vi "Start Logger.vi"(8 "error in (no error)":errorcluster, 11 "Worker in":refnum<class "Worker Actor.lvclass">) -> (0 "error out":errorcluster, 1 "tdms stream out":refnum<k34>, 2 "File Path":path, 3 "Worker out":refnum<class "Worker Actor.lvclass">)   [LabVIEW 2021, in "Worker Actor.lvclass"]
uses:
  Worker Actor.lvclass
  C:/GitHub/LabActor/Template Module/Template Module.lvclass
  Template Module/Template Module.lvclass/Template Module.ctl
  Worker Actor.lvclass/Worker Actor.ctl
  Loggers/Logger/Logger.lvclass/Logger.ctl
  NHMFL_Core/Libraries/File/File Class/File.lvclass/File.ctl
  Template Module/Read Logger.vi
  Read File prefix.vi
  Read Index digits.vi
  Loggers/Logger/Read File.lvclass.vi
  NHMFL_Core/Libraries/File/File Class/Write File Prefix.vi
  NHMFL_Core/Libraries/File/File Class/Write Index digits.vi
  NHMFL_Core/Libraries/File/File Class/Write Root Data Folder.vi
  Loggers/Logger/Write File.lvclass.vi
  Write File Path.vi
  Template Module/Write Logger.vi
  Read Use buffered logger.vi
  Loggers/Logger/Logger.lvclass
  NHMFL_Core/Libraries/File/Metadata/Metadata.lvclass
  NHMFL_Core/Libraries/File/File Class/File.lvclass
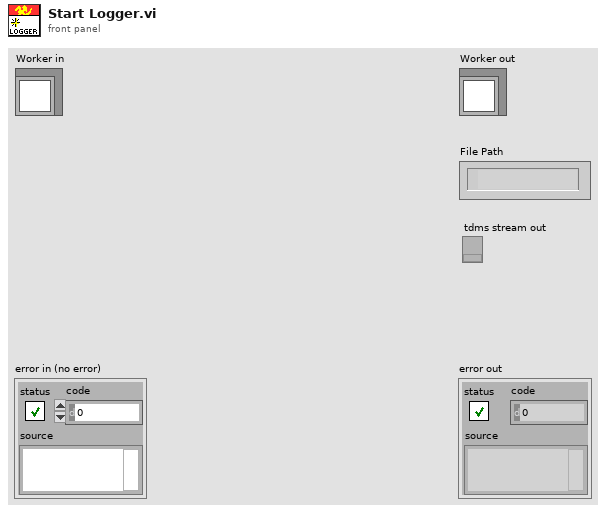
[diagram p1: front panel]
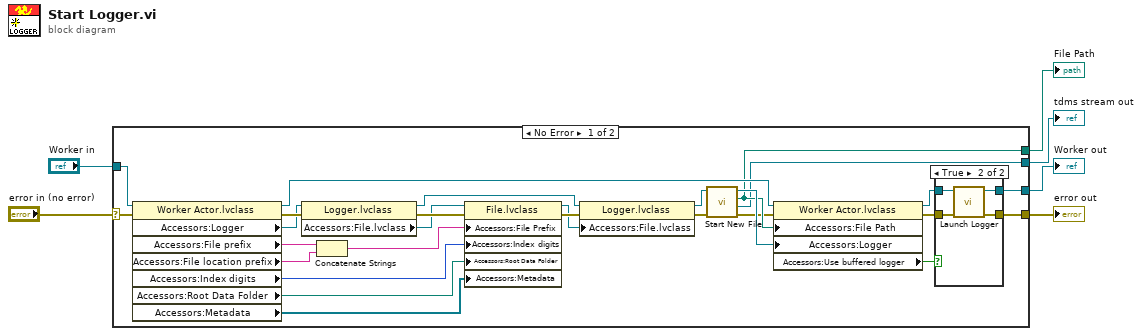
[diagram p0: block diagram]
diagram:
  n1 = case shown="No Error" "error in (no error)" {
    selector: "error in (no error)" -> [w31 w41]
    tunnel: [w14 w41] -> w5
    tunnel: [w13 w40] -> w3
    tunnel: "Worker in" -> [w33 w40]
    tunnel: [w29 _] -> w2
    tunnel: [w9 _] -> w1
    frame No Error {
      n2 = property class="Worker Actor.lvclass"(reference=w33, error in=w31) -> (reference out=w32:refnum<class "Worker Actor.lvclass">, error out=w28:errorcluster, "Accessors:Logger"=w25:refnum<class "Logger.lvclass">, "Accessors:File prefix"=w18:string, "Accessors:File location prefix"=w7:string, "Accessors:Index digits"=w17:i32, "Accessors:Root Data Folder"=w11:path, "Accessors:Metadata"=w10:refnum<class "Metadata.lvclass">[])
      n3 = property class="Logger.lvclass"(reference=w25, error in=w28) -> (reference out=w23:refnum<class "Logger.lvclass">, error out=w26:errorcluster, "Accessors:File.lvclass"=w20:refnum<class "File.lvclass">)
      n4 = Concatenate Strings(w18, w7) -> (w8:string)
      n5 = property class="File.lvclass"(reference=w20, error in=w26, "Accessors:File Prefix"=w8, "Accessors:Index digits"=w17, "Accessors:Root Data Folder"=w11, "Accessors:Metadata"=w10) -> (reference out=w19:refnum<class "File.lvclass">, error out=w21:errorcluster)
      n6 = property class="Logger.lvclass"(reference=w23, error in=w21, "Accessors:File.lvclass"=w19) -> (reference out=w22:refnum<class "Logger.lvclass">, error out=w24:errorcluster)
      n7 = call-dynamic "Start New File.vi"("error in (no error)"=w24, "Logger in"=w22) -> ("error out"=w27:errorcluster, "tdms stream out"=w9:refnum<k34>, "File Path"=w29:path, "Logger out"=w30:refnum<class "Logger.lvclass">)  [unwired: 6 in]
      n8 = property class="Worker Actor.lvclass"(reference=w32, error in=w27, "Accessors:File Path"=w29, "Accessors:Logger"=w30) -> (reference out=w16:refnum<class "Worker Actor.lvclass">, error out=w15:errorcluster, "Accessors:Use buffered logger"=w12:bool)
      n9 = case shown="True" w12 {
        tunnel: w16 -> [w35 w39]
        tunnel: w15 -> [w34 w38]
        tunnel: [w34 w37] -> w14
        tunnel: [w35 w36] -> w13
        frame False {
        }
        frame True {
          n10 = call-dynamic "Launch Logger.vi"("error in (no error)"=w38, "Worker in"=w39) -> ("error out"=w37:errorcluster, "Worker out"=w36:refnum<class "Worker Actor.lvclass">)  [unwired: 8 in]
        }
      }
    }
    frame Error {
    }
  }
  "error out" <- w5
  "Worker out" <- w3
  "File Path" <- w2
  "tdms stream out" <- w1
